vi "Read Execution time.vi"(11 "Test Suite Result In":refnum<class "Test Suite Result.lvclass">) -> (1 "Execution time string":string, 2 "Execution time":dbl, 3 "Test Suite Result Out":refnum<class "Test Suite Result.lvclass">)   [LabVIEW 2020, in "Test Suite Result.lvclass"]
uses:
  Test Suite Result.lvclass
  Test Suite Result.lvclass/Test Suite Result.ctl
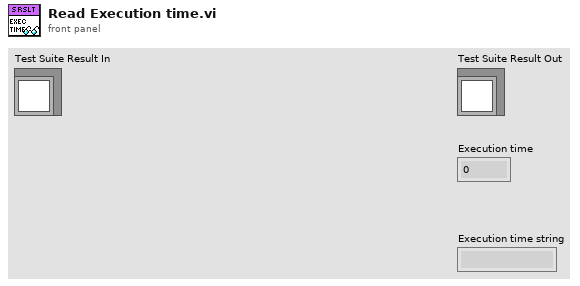
[diagram p1: front panel]
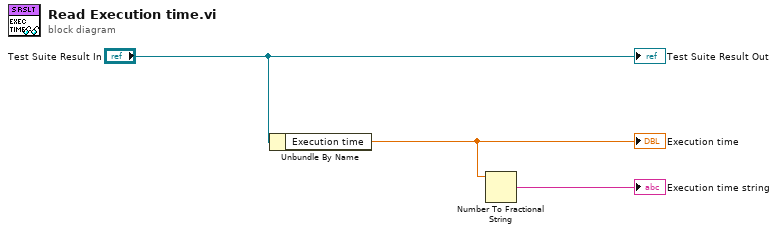
[diagram p0: block diagram]
diagram:
  n1 = Unbundle By Name("Test Suite Result In") -> ("Execution time"=w2:dbl)
  "Execution time" <- w2
  n2 = Number To Fractional String(number=w2) -> (F-format string=→"Execution time string":string)  [unwired: 3 in]
  "Test Suite Result Out" <- "Test Suite Result In"
